vi "PV Software LDO Flags.vi"(11 "HEX Data (U8)":u8[](array[numeric])) -> (3 "LDO Flags":string[](array[string]))   [LabVIEW 2023]
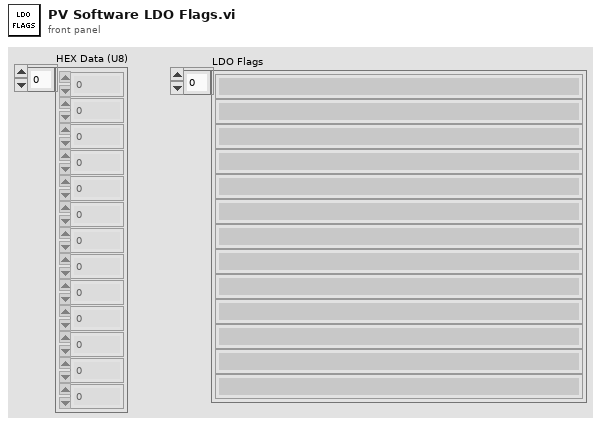
[diagram p1: front panel]
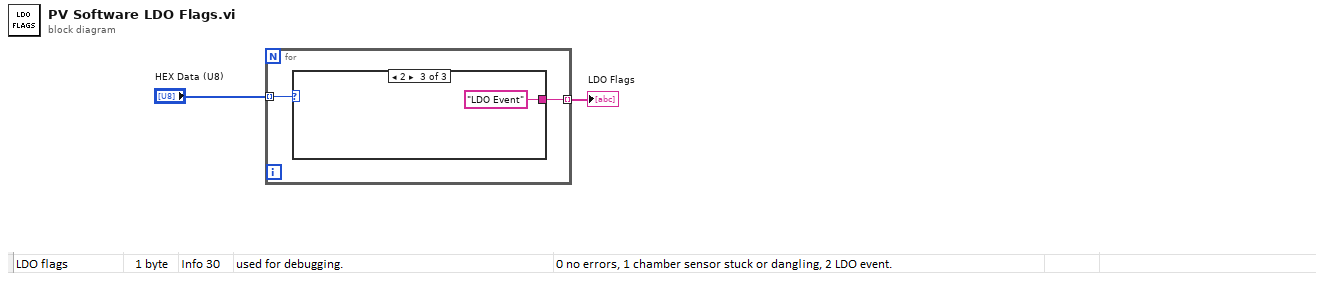
[diagram p0: block diagram]
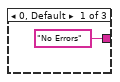
[diagram p2: hidden frame]
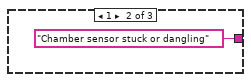
[diagram p3: hidden frame]
diagram:
  n1 = for {
    tunnel: "HEX Data (U8)" -> [w4] mode=indexing
    tunnel: [w3] -> w1 mode=indexing
    n2 = case shown="2" w4 {
      tunnel: ["No Errors" "Chamber sensor stuck or dangling" "LDO Event"] -> w3
      frame 0, Default {
      }
      frame 1 {
      }
      frame 2 {
      }
    }
  }
  "LDO Flags" <- w1
